vi "[SubV]PID.vi"(4 "Left PID gains":T1={"proportional gain (Kc)"=1.0, "integral time (Ti, min)"=0.01, "derivative time (Td, min)"=0.0} {"derivative time (Td, min)" format="%.3f"; "integral time (Ti, min)" format="%.3f"; "proportional gain (Kc)" format="%.3f"}, 6 "Right PID gains":T1={"proportional gain (Kc)"=1.0, "integral time (Ti, min)"=0.01, "derivative time (Td, min)"=0.0} {"derivative time (Td, min)" format="%.3f"; "integral time (Ti, min)" format="%.3f"; "proportional gain (Kc)" format="%.3f"}, 7 "PID Range":cluster{"output high":dbl, "output low":dbl}={"output high"=100.0, "output low"=-100.0} {"output low" format="%.2f"; "output high" format="%.2f"}, 8 "Left Desired Torque":dbl format="%.2f", 9 "Right Desired Torque":dbl format="%.2f", 10 "Left Torque Measured":dbl format="%.2f", 11 "Right Torque Measured":dbl format="%.2f") -> (1 "Left PID Out":dbl format="%.2f", 3 "Right PID Out":dbl format="%.2f")   [LabVIEW 2017]
uses:
  <vilib>/addons/control/pid/pid.llb/PID (DBL).vi
  <vilib>/addons/control/pid/NI_PID_pid.lvlib
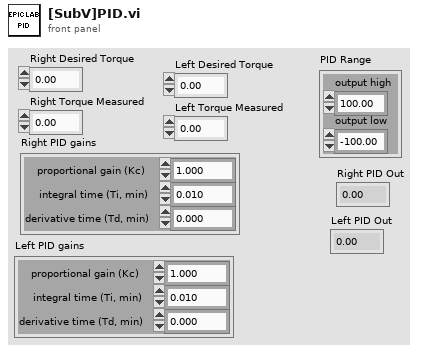
[diagram p1: front panel]
types:
  T1 = cluster{"proportional gain (Kc)":dbl, "integral time (Ti, min)":dbl, "derivative time (Td, min)":dbl}
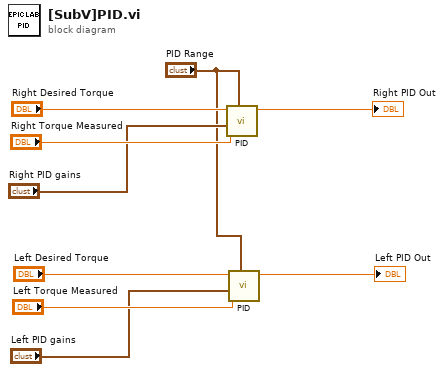
[diagram p0: block diagram]
diagram:
  n1 = call-poly <vilib>:"PID.vi"("output range"="PID Range", "PID gains"="Right PID gains", "process variable"="Right Torque Measured", "setpoint"="Right Desired Torque") -> ("output"=→"Right PID Out":dbl)  [unwired: 6 in, 1 out]
  n2 = call-poly <vilib>:"PID.vi"("output range"="PID Range", "PID gains"="Left PID gains", "process variable"="Left Torque Measured", "setpoint"="Left Desired Torque") -> ("output"=→"Left PID Out":dbl)  [unwired: 6 in, 1 out]
